vi "ShooterMain.vi"(6 "Invert?":bool, 7 "Manual Input":dbl, 8 "Error In":errorcluster, 9 "Reverse":bool, 10 "Forward":bool, 11 "Mode":enum16{"Open", "PID Control", "Manual Control"}(ring)) -> (0 "Error Out":errorcluster, 2 "Output":dbl)   [LabVIEW 2016]
uses:
  <vilib>/Rock Robotics/SystemInterfaces/DIO/FPGA_DIOPWMChannel.ctl
  <vilib>/Rock Robotics/WPI/MotorControl/WPI_MotorControlOpen SPARK.vi
panel:
  # "2017 Shooter Main Control VI\nFRC Team 34"
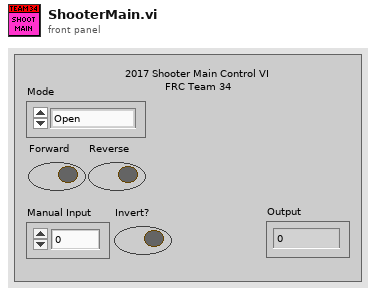
[diagram p1: front panel]
types:
  T1 = typedef "FPGA_DIOPWMChannel.ctl" = enum8{"PWM 0", "PWM 1", "PWM 2", "PWM 3", "PWM 4", "PWM 5", "PWM 6", "PWM 7", "PWM 8", "PWM 9", "PWM MXP 0", "PWM MXP 1", "PWM MXP 2", "PWM MXP 3", "PWM MXP 4", "PWM MXP 5", "PWM MXP 6", "PWM MXP 7", "PWM MXP 8", "PWM MXP 9", "Invalid"}
  T2 = typedef "WPI_MotorControlDeviceRef.ctl" = cluster{"DeviceStatus":errorcluster, "Type":T3, "PWM":cluster{"PWM Channel":T1, "DeadBand":T4}, "CAN":cluster{"Device Number":u8, "SetOutput VI Ref":variant, "GetOutput VI Ref":variant, "Enable VI Ref":variant, "Disable VI Ref":variant, "Data":variant}, "Invert":bool}
  T3 = typedef "WPI_MotorControlType.ctl" = enum16{"PWM", "CAN"}
  T4 = typedef "WPI_PWMDeadband.ctl" = cluster{"Name":string, "maxPositivePwm":i32, "minPositivePwm":i32, "centerPwm":i32, "maxNegativePwm":i32, "minNegativePwm":i32, "angularRange":u16}
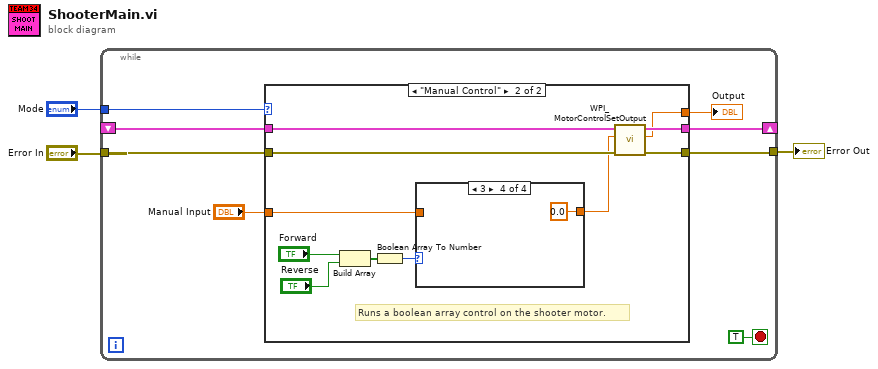
[diagram p0: block diagram]
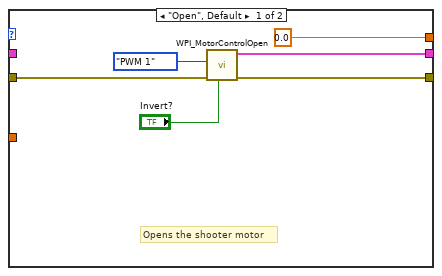
[diagram p2: hidden frame]
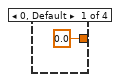
[diagram p3: hidden frame]
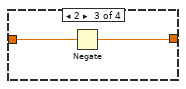
[diagram p5: hidden frame]
diagram:
  n1 = while {
    tunnel: "Mode" -> [w10]
    shift-right: [w9] -> _
    shift-left: _ -> [w8]
    tunnel: "Error In" -> [w6]
    tunnel: [w5] -> w1
    stop <- TRUE stop-if-true
    n2 = case shown="\"Manual Control\"" w10 {
      tunnel: [w17 w27] -> w9
      tunnel: w8 -> [_ w28]
      tunnel: [0.0 ("Motor Output") w26] -> w7
      tunnel: w6 -> [w14 w25]
      tunnel: [w13 w24] -> w5
      tunnel: "Manual Input" -> [_ w20]
      frame "Open", Default {
        # "Opens the shooter motor"
        n3 = call-poly <vilib>:"WPI_MotorControlOpen.vi"("Invert"="Invert?", "error in (no error)"=w14, "PWM Channel"=FPGA_DIOPWMChannel."PWM 1") -> ("error out"=w13:errorcluster, "MotorControlDeviceRef"=w17:T2)  [unwired: 7 in]
      }
      frame "Manual Control" {
        # "Runs a boolean array control on the shooter motor."
        n4 = Build Array("Forward", "Reverse") -> (w21:bool[])
        n5 = Boolean Array To Number(Boolean array=w21) -> (number=w19:u32)
        n6 = case shown="3" w19 {
          tunnel: w20 -> [_ w30 w32 _]
          tunnel: [0.0 ("Manual Input") w30 w31 0.0 ("Manual Input")] -> w18
          frame 0, Default {
          }
          frame 1 {
          }
          frame 2 {
            n7 = Negate(x=w32) -> (-x=w31:dbl)
          }
          frame 3 {
          }
        }
        n8 = call <vilib>:"WPI_MotorControlSetOutput.vi"("error in (no error)"=w25, "Output"=w18, "MotorControlDevRef"=w28) -> ("error out"=w24:errorcluster, "Motor Output"=w26:dbl, "MotorControlDevRef"=w27:T2)  [unwired: 6 in]
      }
    }
    "Output" <- w7
  }
  "Error Out" <- w1
